vi "injector string unpack.vi"(8 "lower limit":dbl, 9 "upper limit":dbl, 11 "Array":string[](array[string])) -> (0 "write data?":bool, 1 "data out":T1, 2 "mass flow/setpoint":cluster{"[4]":dbl, "[5]":dbl}, 3 "pressure/temp":cluster{"[1]":dbl, "[2]":dbl}, 4 "current time":timestamp, 5 "Waveform":waveform(dbl), 6 "Temp In Range?":bool=TRUE)   [LabVIEW 2016]
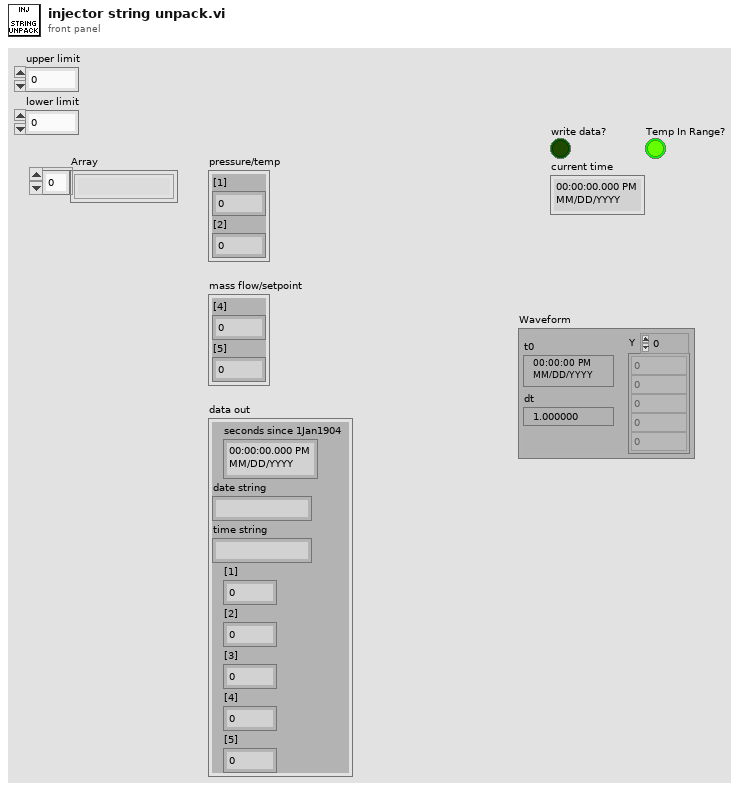
[diagram p1: front panel]
types:
  T1 = cluster{"seconds since 1Jan1904":timestamp, "date string":string, "time string":string, "[1]":dbl, "[2]":dbl, "[3]":dbl, "[4]":dbl, "[5]":dbl}
  T2 = cluster{"[0]":dbl, "[1]":dbl, "[2]":dbl, "[3]":dbl, "[4]":dbl, "[5]":dbl, "[6]":dbl, "[7]":dbl, "[8]":dbl}
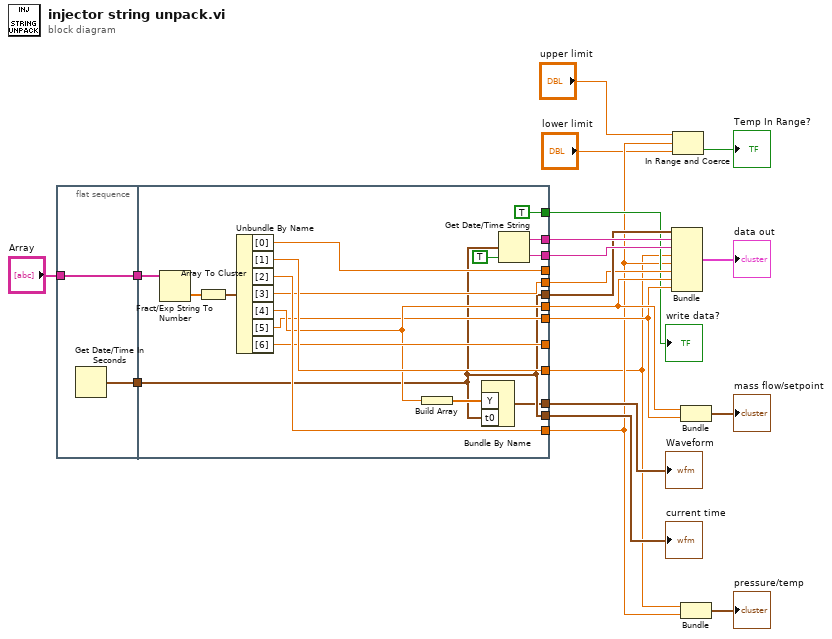
[diagram p0: block diagram]
diagram:
  n1 = flat-sequence {
    tunnel: "Array" -> [w22]
    tunnel: [w22] -> w20
    tunnel: [w21] -> w19
    tunnel: w20 -> [w35]
    tunnel: w19 -> [w24]
    tunnel: [w24] -> w15
    tunnel: [w38] -> w16
    tunnel: [w37] -> w17
    tunnel: [w33] -> _
    tunnel: [w32] -> w3
    tunnel: [w31] -> w5
    tunnel: [w30] -> w14
    tunnel: [w27] -> w13
    tunnel: [w26] -> w12
    tunnel: [w29] -> _
    tunnel: [TRUE] -> w8
    tunnel: [w24] -> w7
    tunnel: [w23] -> w6
    frame #0 {
      n2 = Get Date/Time In Seconds() -> (seconds since 1Jan1904=w21:timestamp)
    }
    frame #1 {
      n3 = Fract/Exp String To Number(string=w35) -> (number=w34:dbl[])  [unwired: 3 in, 1 out]
      n4 = Array To Cluster(array=w34) -> (cluster=w36:T2)
      n5 = Unbundle By Name(w36) -> ("[0]"=w33:dbl, "[1]"=w32:dbl, "[2]"=w31:dbl, "[3]"=w30:dbl, "[4]"=w27:dbl, "[5]"=w26:dbl, "[6]"=w29:dbl)
      n6 = Build Array(w27) -> (w25:dbl[])
      n7 = Bundle By Name("Y"=w25, "t0"=w24) -> (w23:waveform(dbl))  [unwired: 1 in]
      n8 = Get Date/Time String(seconds (now)=w24, want seconds? (F)=TRUE) -> (date string=w38:string, time string=w37:string)  [unwired: 1 in]
    }
  }
  n9 = Bundle("seconds since 1Jan1904"=w15, "date string"=w16, "time string"=w17, "[1]"=w3, "[2]"=w5, "[3]"=w14, "[4]"=w13, "[5]"=w12) -> (→"data out":T1)  [unwired: 1 in]
  n10 = In Range and Coerce(upper limit="upper limit", x=w5, lower limit="lower limit") -> (In Range?=→"Temp In Range?":bool)  [unwired: 1 out]
  n11 = Bundle("[4]"=w13, "[5]"=w12) -> (→"mass flow/setpoint":cluster{"[4]":dbl, "[5]":dbl})  [unwired: 1 in]
  n12 = Bundle("[1]"=w3, "[2]"=w5) -> (→"pressure/temp":cluster{"[1]":dbl, "[2]":dbl})  [unwired: 1 in]
  "write data?" <- w8
  "current time" <- w7
  "Waveform" <- w6
